vi "test Mock Transceiver With Transmit Error.vi"(8 "error in (no error)":errorcluster, 11 "TestCase in":refnum<class "Transceiver Test Cases.lvclass">) -> (0 "error out":errorcluster, 3 "TestCase out":refnum<class "Transceiver Test Cases.lvclass">)   [LabVIEW 2017, in "Transceiver Test Cases.lvclass"]
uses:
  Transceiver Test Cases.lvclass
  Configuration/Public/Controls/DSF Engine Transfer Group Configuration.ctl
  Configuration/Public/Controls/DSF Direction.ctl
  Configuration/Public/Controls/DSF Timing Info.ctl
  Configuration/Public/Controls/DSF Engine Transfer Configuration.ctl
  Configuration/Public/Controls/DSF Byte Order.ctl
  Configuration/Public/Controls/DSF Engine Channel Configuration.ctl
  Configuration/Public/Controls/DSF Data Type.ctl
  Configuration/Public/Controls/DSF Settings Info.ctl
  MockTransceiver.lvclass
  Engine/Classes/Transfer Group/Transfer Group.lvclass
  DSF Core.lvlib
  <vilib>/addons/_JKI Toolkits/VI Tester/TestCase.llb/TestCase.lvclass
  C:/Program Files (x86)/National Instruments/LabVIEW 2017/vi.lib/addons/_JKI Toolkits/VI Tester/TestCase.llb/TestCase.lvclass
panel:
  out "expected error":errorcluster
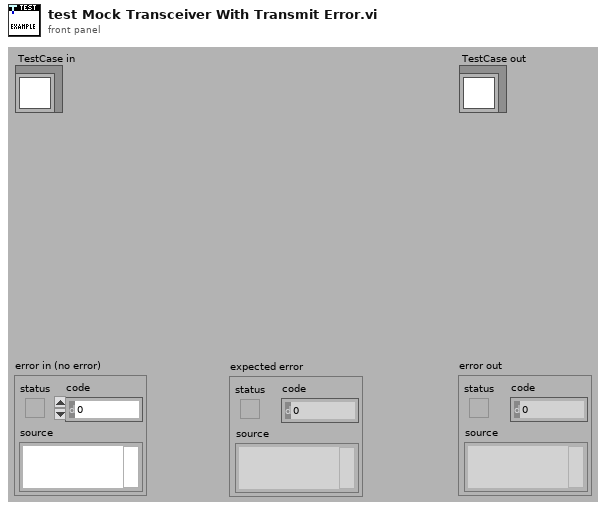
[diagram p1: front panel]
types:
  T1 = typedef "DSF Core.lvlib/DSF Settings Info.ctl" = cluster{"key":string, "value":string}[]
  T2 = typedef "DSF Core.lvlib/DSF Engine Transfer Group Configuration.ctl" = cluster{"name":string, "direction":T3, "cycle timing":T4, "Transfers":T5[], "settings":T1}
  T3 = typedef "DSF Core.lvlib/DSF Direction.ctl" = enum8{"Tx", "Rx"}
  T4 = typedef "DSF Core.lvlib/DSF Timing Info.ctl" = cluster{"priority":u64, "decimation":u64, "offset":u64}
  T5 = typedef "DSF Core.lvlib/DSF Engine Transfer Configuration.ctl" = cluster{"name":string, "byte order":T6, "channel configurations":T7[], "settings":T1}
  T6 = typedef "DSF Core.lvlib/DSF Byte Order.ctl" = enum8{"big-endian", "little-endian"}
  T7 = typedef "DSF Core.lvlib/DSF Engine Channel Configuration.ctl" = cluster{"engine offset":u64, "name":string, "data type":T8, "count":u64, "buffer offset":u64}
  T8 = typedef "DSF Core.lvlib/DSF Data Type.ctl" = enum8{"Bool", "SGL", "DBL", "I8", "I16", "I32", "I64", "U8", "U16", "U32", "U64"}
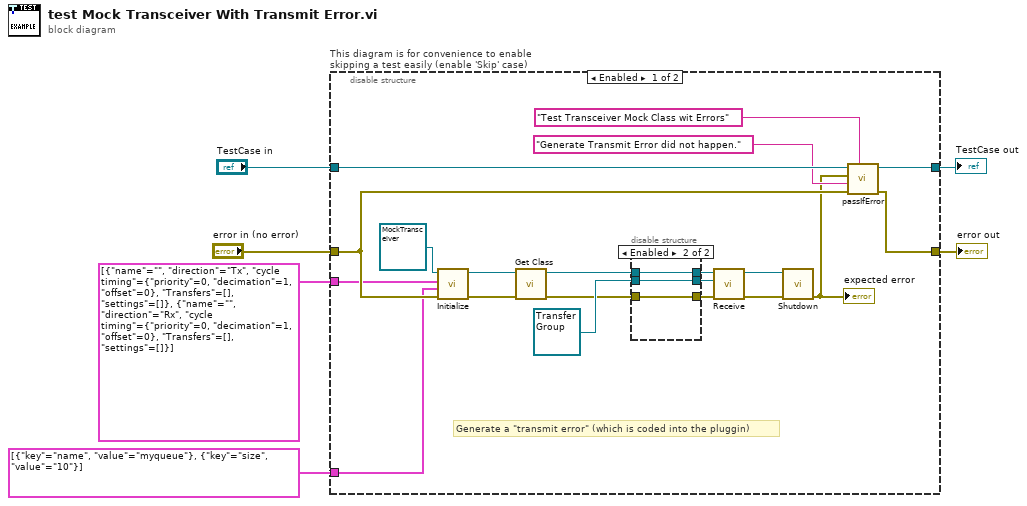
[diagram p0: block diagram]
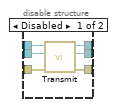
[diagram p2: hidden frame]
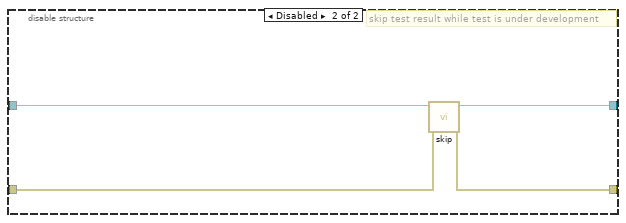
[diagram p3: hidden frame]
diagram:
  n1 = disable-structure "This diagram is for convenience to enable skipping a test easily (enable 'Skip' case)" shown="Enabled" {
    disable-tunnel: "TestCase in" -> [w26 w39]
    disable-tunnel: [w25 w37] -> w5
    disable-tunnel: [w7 w38] -> w4
    disable-tunnel: "error in (no error)" -> [w24 w36]
    disable-tunnel: T2[] [{"name"="", "direction"=enum."Tx", "cycle timing"={"priority"=0, "decimation"=1, "offset"=0}, "Transfers"=[], "settings"=[]}, {"name"="", "direction"=enum."Rx", "cycle timing"={"priority"=0, "decimation"=1, "offset"=0}, "Transfers"=[], "settings"=[]}] ("Transfer Groups Configurations") -> [w13 _]
    disable-tunnel: T1 [{"key"="name", "value"="myqueue"}, {"key"="size", "value"="10"}] ("transceiver settings") -> [w12 _]
    frame Enabled {
      # "Generate a \"transmit error\" (which is coded into the pluggin)"
      n2 = call-dynamic "Initialize.vi"("error in (no error)"=w24, "transceiver settings"=w12, "Transfer Groups Configurations"=w13, "MockTransceiver in"=refnum<class "MockTransceiver.lvclass"> refnum) -> ("error out"=w14:errorcluster, "MockTransceiver out"=w15:refnum<class "MockTransceiver.lvclass">)  [unwired: 6 in]
      n3 = call-dynamic "Get Class.vi"("error in (no error)"=w14, "MockTransceiver in"=w15) -> ("error out"=w16:errorcluster, "MockTransceiver out"=w17:refnum<class "MockTransceiver.lvclass">)  [unwired: 7 in, 1 out]
      n4 = disable-structure shown="Enabled" {
        disable-tunnel: refnum<class "Transfer Group.lvclass"> refnum ("Transfer Group in") -> [w32 w34]
        disable-tunnel: [w31 w35] -> w20
        disable-tunnel: [w30 w34] -> w19
        disable-tunnel: [w29 w33] -> w18
        disable-tunnel: w17 -> [w28 w35]
        disable-tunnel: w16 -> [w27 w33]
        frame Disabled {
          n5 = call-dynamic "Transmit.vi"("error in (no error)"=w27, "Transfer Group in"=w32, "MockTransceiver in"=w28) -> ("error out"=w29:errorcluster, "Transfer Group out"=w30:refnum<class "Transfer Group.lvclass">, "MockTransceiver out"=w31:refnum<class "MockTransceiver.lvclass">)  [unwired: 6 in]
        }
        frame Enabled {
        }
      }
      n6 = call-dynamic "Receive.vi"("error in (no error)"=w18, "Transfer Group in"=w19, "MockTransceiver in"=w20) -> ("error out"=w9:errorcluster, "MockTransceiver out"=w10:refnum<class "MockTransceiver.lvclass">)  [unwired: 6 in, 1 out]
      n7 = call-dynamic "Shutdown.vi"("error in (no error)"=w9, "MockTransceiver in"=w10) -> ("error out"=w8:errorcluster)  [unwired: 8 in, 1 out]
      "expected error" <- w8
      n8 = call-dynamic "passIfError.vi"("custom report message (\"\")"="Test Transceiver Mock Class wit Errors" ("custom report message (\"\")"), "error in (no error)"=w24, "task (\"\")"="Generate Transmit Error did not happen." ("custom report message (\"\")"), "error"=w8, "TestCase in"=w26) -> ("error out"=w7:errorcluster, "TestCase out"=w25:refnum<class "Transceiver Test Cases.lvclass">)  [unwired: 5 in]
    }
    frame Disabled {
      # "skip test result while test is under development"
      n9 = call <vilib>:"skip.vi"("error in (no error)"=w36, "TestCase in"=w39) -> ("error out"=w38:errorcluster, "TestCase out"=w37:refnum<class "Transceiver Test Cases.lvclass">)  [unwired: 8 in]
    }
  }
  "error out" <- w4
  "TestCase out" <- w5
